vi "UPDATE_Export_Data_From_TXT_figures_v1.3-Sh.vi"() -> ()   [LabVIEW 2018]
uses:
  <vilib>/Native 3D Graph/xcontrol/3DPC_SurfacePlot.xctl
panel:
  in  "Длина":dbl
  in  "Ширина":dbl
  out "XY Graph":T1(graph)
  out "3D Graph":refnum<class "Base Datatype.lvclass">[](xcontrol)
  out "array":dbl[][](array[numeric])
  in  "Open":bool
  in  "Выбор файла":path
  # "Z"
  # "№ отм."
  # "X"
  # "Y"
  # "Настройки прямоугольника:"
  # "После ввода значений, нажмите \"Загрузить\""
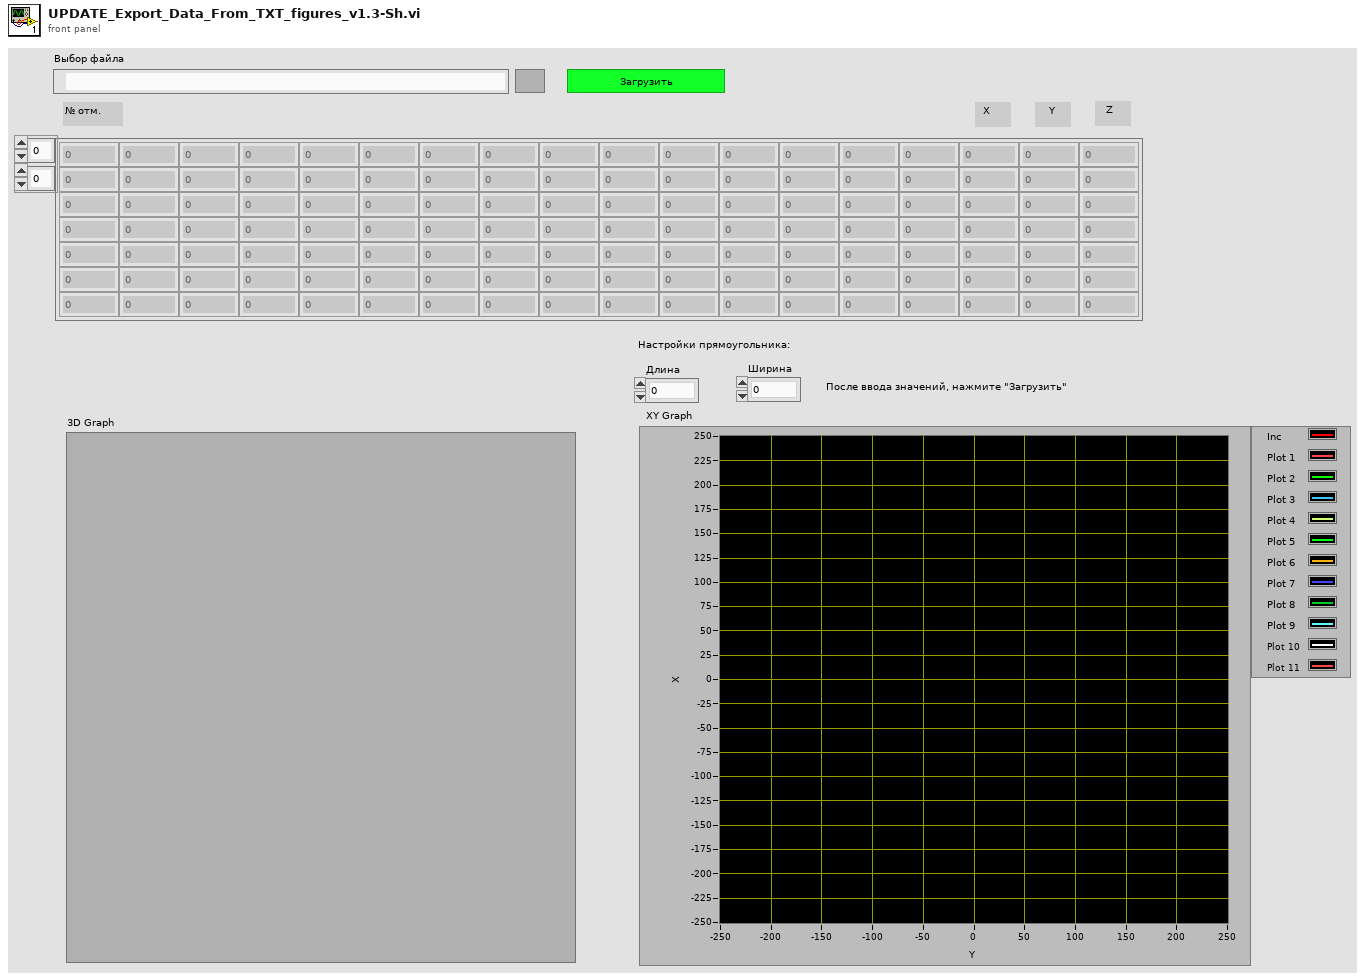
[diagram p1: front panel]
types:
  T1 = cluster{"type (empty)":dbl[], "type (empty)":dbl[]}[]
  T2 = cluster{"type (empty)":dbl[], "type (empty)":dbl[]}
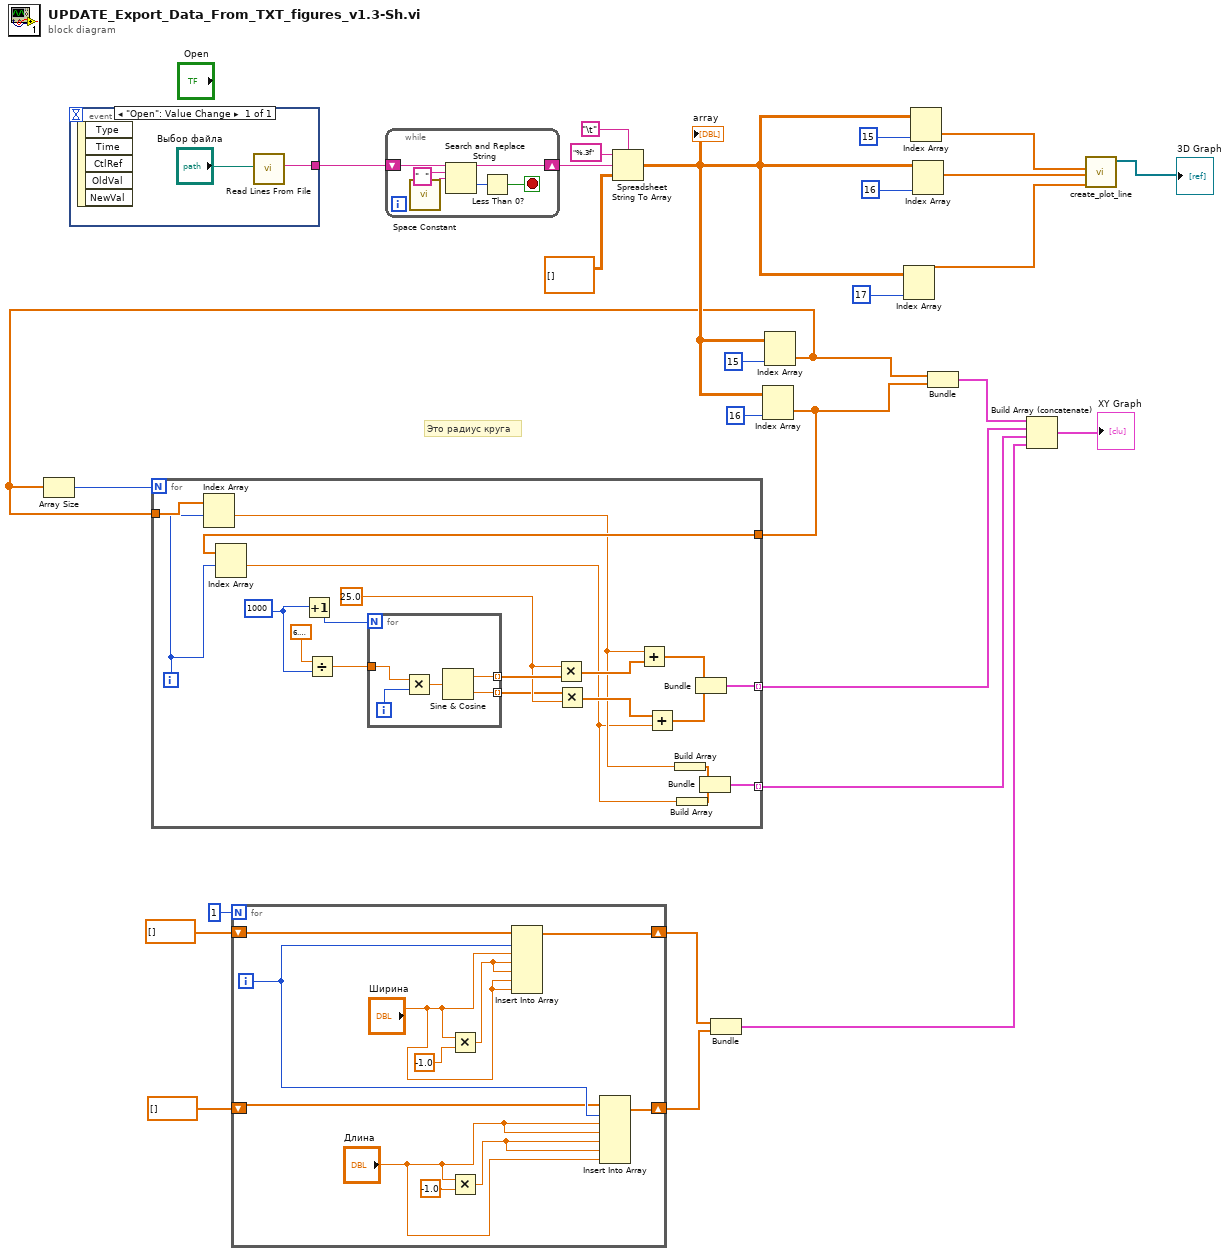
[diagram p0: block diagram]
diagram:
  # "Это радиус круга"
  n1 = event shown="[0] \"Open\": Value Change" {
    selector: _ -> [_]
    dyn-events: _ -> [_]
    timeout: _ -> [_]
    tunnel: [w30] -> w24
    event "Open": Value Change {
      n2 = event-data() -> ()  [unwired: 1 in, 5 out]
      n3 = call <vilib>:"Read Lines From File.vi"("file path (dialog if empty)"="Выбор файла") -> ("line string"=w30:string)  [unwired: 1 in, 7 out]
    }
  }
  n4 = for {
    N: 1 -> [_]
    shift-right: [w35] -> w1
    shift-left: dbl[] [] ("Array 5") -> [w36]
    shift-right: [w33] -> w3
    shift-left: dbl[] [] ("Array 7") -> [w32]
    i -> [w34]
    n5 = Multiply(x="Ширина", y=-1.0) -> (x*y=w40:dbl)
    n6 = Multiply(x="Длина", y=-1.0) -> (x*y=w37:dbl)
    n7 = Insert Into Array(array=w36, index=w34, new element #1="Ширина", new element #2=w40, new element #3=w40, new element #4="Ширина", new element #5="Ширина") -> (w35:dbl[])
    n8 = Insert Into Array(array=w32, index=w34, new element #1="Длина", new element #2="Длина", new element #3=w37, new element #4=w37, new element #5="Длина") -> (w33:dbl[])
  }
  n9 = while {
    shift-right: [w44] -> w26
    shift-left: w24 -> [w47]
    stop <- w42 stop-if-true
    n10 = call <vilib>:"Space Constant.vi"() -> ("String"=w45:string)
    n11 = Search and Replace String(input string=w47, search string="  ", replace string=w45) -> (result string=w44:string, offset past replacement=w43:i32)  [unwired: 1 in, 6 out]
    n12 = Less Than 0?(x=w43) -> (x < 0?=w42:bool)
  }
  n13 = Spreadsheet String To Array(delimiter (Tab)="\t", format string="%.3f" ("format (%.3f)"), spreadsheet string=w26, array type (2D Dbl)=dbl[][] [] ("type (empty)")) -> (array=w16:dbl[][])
  "array" <- w16
  n14 = Bundle("Array 5"=w1, "Array 7"=w3) -> (w2:cluster{"Array 5":dbl[], "Array 7":dbl[]})  [unwired: 1 in]
  n15 = Index Array(array=w16, index (col)=16) -> (element=w10:dbl[])  [unwired: 1 in]
  n16 = Index Array(array=w16, index (col)=15) -> (element=w12:dbl[])  [unwired: 1 in]
  n17 = Array Size(array=w12) -> (size(s)=w9:i32)
  n18 = for {
    N: w9 -> [_]
    tunnel: w12 -> [w66]
    tunnel: w10 -> [w67]
    tunnel: [w50] -> w8 mode=indexing
    tunnel: [w49] -> w7 mode=indexing
    i -> [w65]
    w53 = 25.0
    w57 = 1000 ("x")
    w69 = 1000 ("N")
    n19 = Increment(x=w69) -> ()  [unwired: 1 out]
    n20 = Divide(x=6.283185307179586, y=w69) -> ()  [unwired: 1 out]
    n21 = Index Array(array=w66, index #1=w65) -> (element #1=w52:dbl)  [unwired: 1 in, 1 out]
    n22 = Index Array(array=w67, index #1=w65) -> (element #1=w51:dbl)  [unwired: 1 in, 1 out]
    n23 = Increment(x=w57) -> (x+1=w63:i32)
    n24 = Divide(x=6.283185307179586, y=w57) -> (x/y=w56:dbl)
    n25 = for {
      N: w63 -> [_]
      tunnel: w56 -> [w74]
      tunnel: [w71] -> w48 mode=indexing
      tunnel: [w70] -> w64 mode=indexing
      i -> [w73]
      n26 = Multiply(x=w74, y=w73) -> (x*y=w72:dbl)
      n27 = Sine & Cosine(0:w72) -> (1:w70:dbl, 2:w71:dbl)
    }
    n28 = Multiply(x=w53, y=w64) -> (x*y=w58:dbl[])
    n29 = Multiply(x=w48, y=w53) -> (x*y=w60:dbl[])
    n30 = Add(x=w52, y=w58) -> (x+y=w61:dbl[])
    n31 = Add(x=w60, y=w51) -> (x+y=w59:dbl[])
    n32 = Build Array(w52) -> (w55:dbl[])
    n33 = Build Array(w51) -> (w54:dbl[])
    n34 = Bundle(w61, w59) -> (w50:cluster{dbl[], dbl[]})  [unwired: 1 in]
    n35 = Bundle(w55, w54) -> (w49:cluster{dbl[], dbl[]})  [unwired: 1 in]
  }
  n36 = Index Array(array=w16, index (col)=17) -> (element=w11:dbl[])  [unwired: 1 in]
  n37 = Index Array(array=w16, index (col)=15) -> (element=w18:dbl[])  [unwired: 1 in]
  n38 = Index Array(array=w16, index (col)=16) -> (element=w19:dbl[])  [unwired: 1 in]
  n39 = Bundle("type (empty)"=w12, "type (empty)"=w10) -> (w13:T2)  [unwired: 1 in]
  n40 = Build Array (concatenate)(w13, w8, w7, w2) -> (→"XY Graph":cluster{"Array 5":dbl[], "Array 7":dbl[]}[])
  n41 = call <vilib>:"create_plot_line.vi"("z vector"=w11, "y vector"=w19, "x vector"=w18) -> ("plots out"=→"3D Graph":refnum<class "Base Datatype.lvclass">[])  [unwired: 2 in, 6 out]
